vi "AOD Control - debugging(host).vi"() -> ()   [LabVIEW 2009]
uses:
  <vilib>/userdefined/High Color/nirio_resource_hc.ctl
  <vilib>/rvi/interface/nirviOpenFPGA/nirviOpenFPGA.xnode
  FPGA Bitfiles/AOD Control.lvproj_FPGA Target_AOD Control (FPGA)~D2.lvbitx
  AOD Control (FPGA).vi
  <vilib>/rvi/interface/RandomDataEmulation/nirviRandomDataOpen.vi
  <vilib>/rvi/interface/nirviOpenFPGA/nirviOpenFPGA.ctl
  <vilib>/rvi/interface/nirviOpenFPGA/nirviopenstate.ctl
  <vilib>/picture/picture.llb/imagedata.ctl
  <vilib>/rvi/interface/common/nirviIntfCommonState.ctl
  <vilib>/rvi/interface/common/nirviIntfModes.ctl
  C:/Program Files/National Instruments/LabVIEW 2009/resource/RVI/emulation/niLvFpgaEmulationMode.ctl
  <vilib>/eio/XNode/Errors/EIOXNodeErrorStruct.ctl
  <vilib>/eio/XNode/Errors/EIOXNodeInternalErrorTypes.ctl
  <vilib>/eio/XNode/Errors/EIOXNodeUserErrorTypes.ctl
  <vilib>/XNodeSupport/XNodeRect32.ctl
  <vilib>/XNodeSupport/XNodeInt.ctl
  <vilib>/XNodeSupport/XNodeTerms.ctl
  <vilib>/XNodeSupport/XNodeTerm.ctl
  <vilib>/XNodeSupport/XNodeString.ctl
  <vilib>/XNodeSupport/XNodeVariant.ctl
  <vilib>/XNodeSupport/XNodeBool.ctl
  <vilib>/rvi/interface/nirviMethod/nirviMethod.xnode
  <vilib>/FPGA/interface/niFpgaViExecutionMode.ctl
  <vilib>/rvi/errors/niLvFpgaMergeErrorWithErrorCode.vi
  <vilib>/rvi/interface/RandomDataEmulation/nirviRandomDataRunMethod.vi
  <vilib>/rvi/interface/RandomDataEmulation/nirviRandomDataDMAMethods.vi
  <vilib>/rvi/interface/common/niFpgaNodeNameForErrorReporting.ctl
  <vilib>/rvi/interface/nirviReadWriteControl/nirviReadWriteControl.xnode
  <vilib>/Waveform/DWDTOps.llb/DWDT Binary U16 to Digital.vi
  <vilib>/XNodeSupport/NI_XNodeSupport.lvlib
panel:
  in  "TriggerAcq":bool=TRUE
  out "State":T1(ring)
  out "SerialError":bool
  in  "Abort":bool
  out "Acquire":bool
  out "SampleCount":i16
  in  "AcqDivider":i32=10
  in  "Downsample":i32=160
  in  "Reset":bool
  in  "SclkDivider":u32=40
  in  "Pause":u32
  in  "P":bool
  in  "Volume Scan":bool
  in  "Scan Settings":T2={"XStart"=-200000000, "XEnd"=200000000, "XInc"=20000000, "YStart"=-200000000, "YEnd"=200000000, "YInc"=20000000, "ZStart"=-40000, "ZEnd"=40000, "ZInc"=400}
  out "PointTime":u32
  out "NumReps":i32
  out "NumPoints":i32
  out "Read Point":cluster{"X":i32, "Y":i32, "Z":i32}
  out "PointNum":u32
  out "Sequencing error":bool
  out "Count":i32
  in  "Points":i32[][](array[numeric])
  in  "Scans":i32
  in  "Scan":bool
  out "Write count":i32
  out "Written":cluster{"Address":u8, "Value":u32}[](array[cluster]) {"Address" format="%x"; "Value" format="%x"}
  in  "Write Point":bool
  in  "Write Registers":cluster{"Address":u8, "Value":u32}[](array[cluster])=[{"Address"=0, "Value"=240}, {"Address"=1, "Value"=13762592}, {"Address"=2, "Value"=32768}, {"Address"=3, "Value"=8413952}, {"Address"=4, "Value"=0}, {"Address"=5, "Value"=0}, {"Address"=6, "Value"=1023}, {"Address"=7, "Value"=257}, {"Address"=8, "Value"=21}, {"Address"=0, "Value"=246}] {"Address" format="%x"; "Value" format="%x"}
  in  "UpdatesPerPoint":u32=2000
  in  "Write Point":cluster{"X":i32, "Y":i32, "Z":i32}
  in  "Samples":u32=1000
  in  "WriteSize":enum16{"1", "2", "4"}(ring)
  in  "Loopback delay":u32=4
  out "ControlSignals":digitalwaveform(graph)
  out "Elements Remaining":u32
  in  "Stop":bool
  in  "Write Register":bool
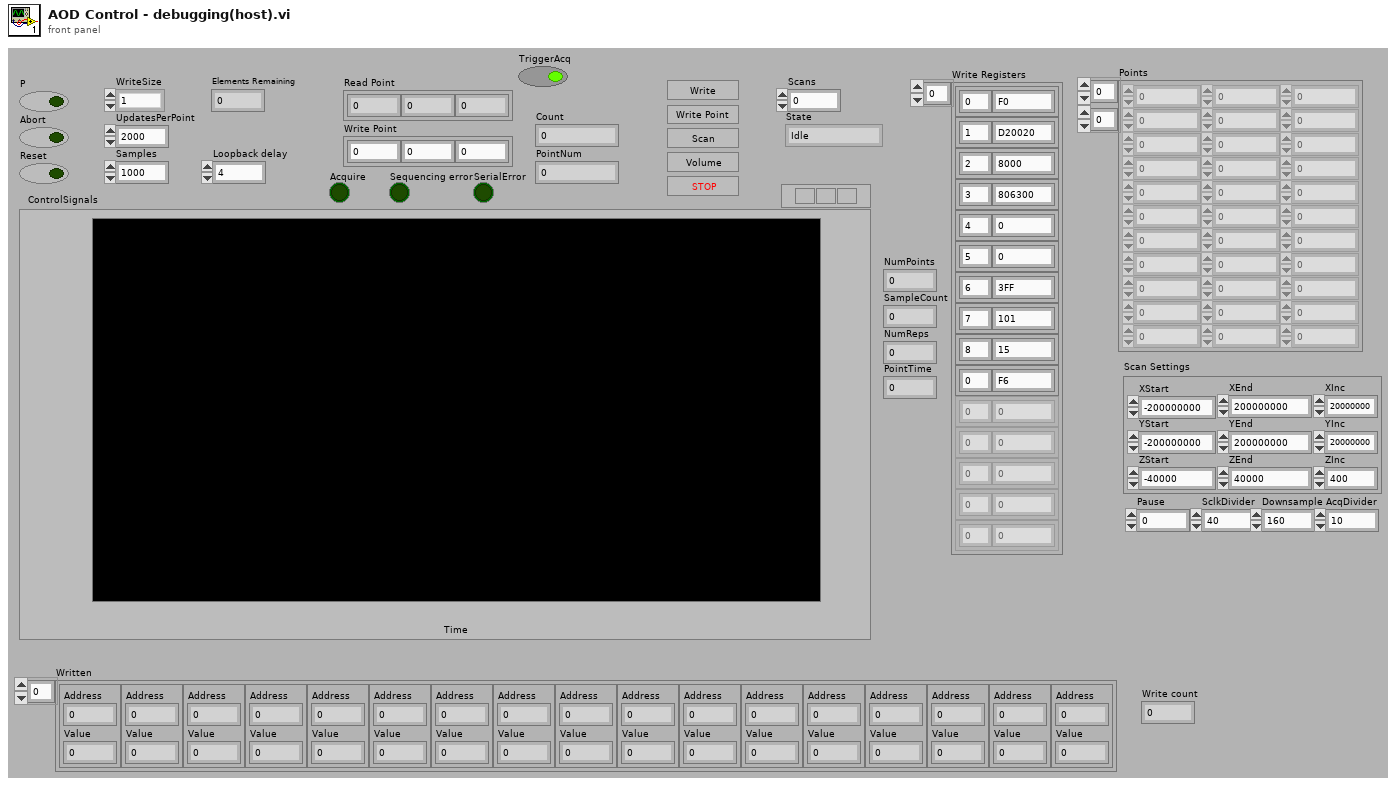
[diagram p1: front panel]
types:
  T1 = enum16{"Idle", "Write Registers", "Receive Points", "Prepare Volume", "Arm Scan", "Scan Points"}
  T2 = cluster{"XStart":i32, "XEnd":i32, "XInc":i32, "YStart":i32, "YEnd":i32, "YInc":i32, "ZStart":i32, "ZEnd":i32, "ZInc":i32}
  T3 = typedef "nirio_resource_hc.ctl" = tag
  T4 = typedef "niFpgaViExecutionMode.ctl" = enum16{"FPGA Target", "Development Computer with Simulated I/O", "Development Computer with Real I/O"}
  T5 = enum16{"Idle", "Write Registers", "Receive Points", "Scan Points"}
  T6 = typedef "niFpgaNodeNameForErrorReporting.ctl" = enum16{"Open FPGA VI Reference", "Read/Write Control", "Invoke Method: Abort", "Invoke Method: Acknowledge IRQ", "Invoke Method: Download", "Invoke Method: FIFO.Configure", "Invoke Method: FIFO.Read", "Invoke Method: FIFO.Start", "Invoke Method: FIFO.Stop", "Invoke Method: FIFO.Write", "Invoke Method: Reset", "Invoke Method: Run", "Invoke Method: Wait on IRQ", "Close FPGA VI Reference"}
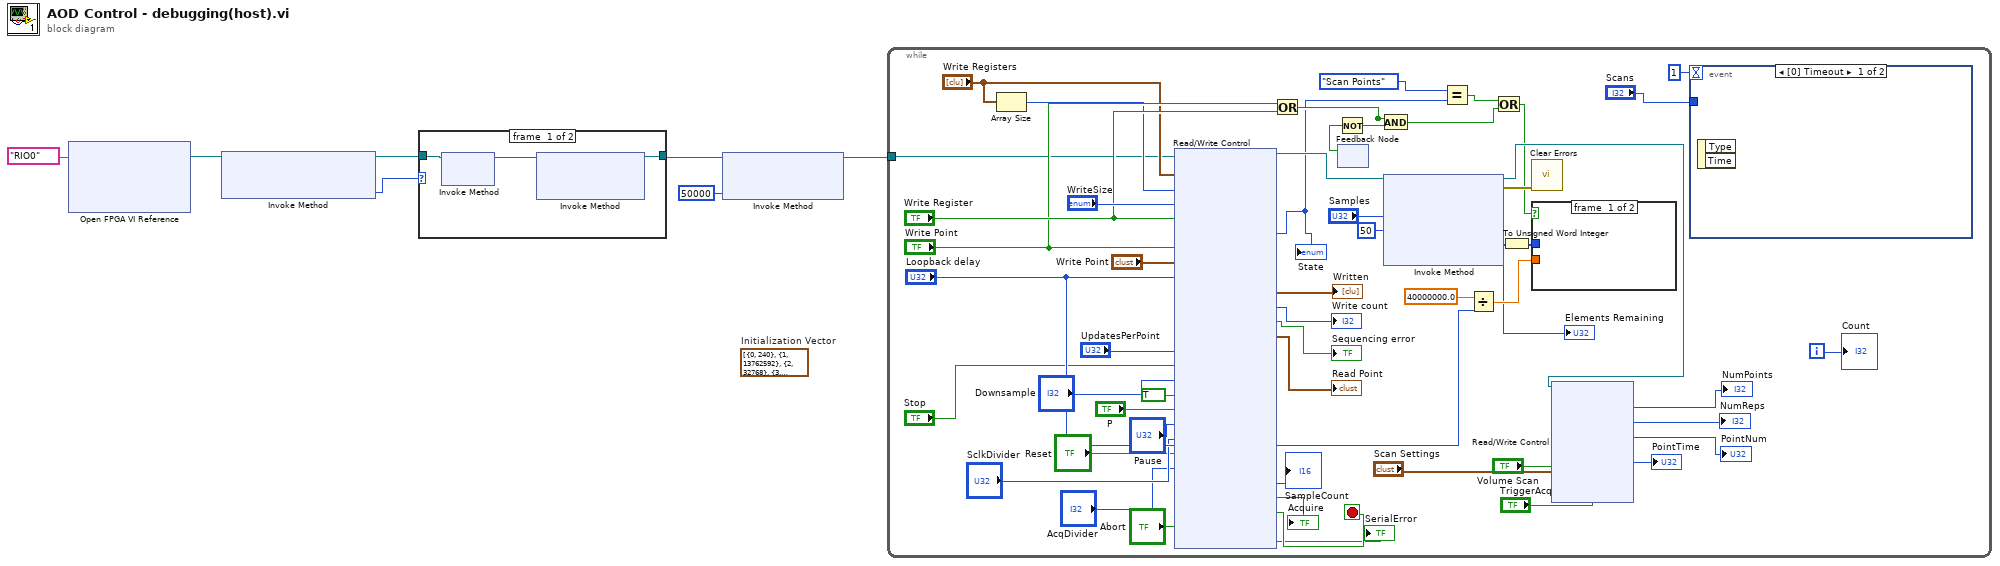
[diagram p0: block diagram]
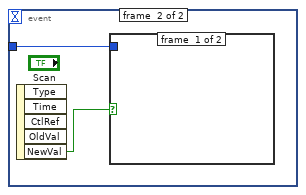
[diagram p3: hidden frame]
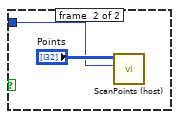
[diagram p4: hidden frame]
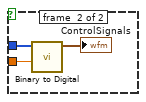
[diagram p5: hidden frame]
diagram:
  (unwired) cluster{"Address":u8, "Value":u32}[] [{"Address"=0, "Value"=240}, {"Address"=1, "Value"=13762592}, {"Address"=2, "Value"=32768}, {"Address"=3, "Value"=8413952}, {"Address"=4, "Value"=0}, {"Address"=5, "Value"=0}, {"Address"=6, "Value"=1023}, {"Address"=7, "Value"=257}, {"Address"=8, "Value"=21}, {"Address"=0, "Value"=246}]  # Initialization Vector
  n1 = xnode "Open FPGA VI Reference"("resource name"=T3 "RIO0") -> ("FPGA VI Reference Out"=w4:refnum<k20>)  [unwired: 1 in, 1 out]
  n2 = xnode "Invoke Method"("FPGA VI Reference In"=w4) -> ("FPGA VI Reference Out"=w2:refnum<k20>, "FPGA VI Execution Mode"=w3:T4)  [unwired: 1 in, 1 out]
  n3 = case shown="\"FPGA Target\", Default" w3 {
    tunnel: [w8 w24] -> w5
    tunnel: w2 -> [w9 w24]
    frame #0 {
      n4 = xnode "Invoke Method"("FPGA VI Reference In"=w9) -> ("FPGA VI Reference Out"=w10:refnum<k20>)  [unwired: 1 in, 1 out]
      n5 = xnode "Invoke Method"("FPGA VI Reference In"=w10) -> ("FPGA VI Reference Out"=w8:refnum<k20>)  [unwired: 2 in, 1 out]
    }
    frame #1 {
    }
  }
  n6 = xnode "Invoke Method"("FPGA VI Reference In"=w5, "Depth"=u32 50000) -> ("FPGA VI Reference Out"=w6:refnum<k20>)  [unwired: 1 in, 1 out]
  n7 = while {
    tunnel: w6 -> [w61]
    i -> [w60]
    stop <- w30 stop-if-true
    n8 = Array Size(array="Write Registers") -> (size(s)=w64:i32)
    n9 = xnode "Read/Write Control"("FPGA VI Reference In"=w61, "Register Writes"="Write Registers", "Number Registers"=w64, "WriteSize"="WriteSize", "Write Register"="Write Register", "Write Point"="Write Point", "Point"="Write Point", "Loopback delay"="Loopback delay", "UpdatesPerPoint"="UpdatesPerPoint", "stop"="Stop", "Downsample"="Downsample", "Loopback"=TRUE, "P"="P", "Pause"="Pause", "SclkDivider"="SclkDivider", "Reset"="Reset", "AcqDivider"="AcqDivider", "Abort"="Abort") -> ("FPGA VI Reference Out"=w70:refnum<k20>, "State"=w27:T1, "Written"=→"Written":cluster{"Address":u8, "Value":u32}[], "Write count"=→"Write count":i32, "Sequencing error"=→"Sequencing error":bool, "Point"=→"Read Point":cluster{"X":i32, "Y":i32, "Z":i32}, "SampleCount"=→"SampleCount":u32, "Acquire"=→"Acquire":bool, "Stopped"=w30:bool, "SerialError"=→"SerialError":bool)  [unwired: 1 in, 1 out]
    "State" <- w27
    n10 = Or(x="Write Point", y="Write Register") -> (x .or. y?=w68:bool)
    n11 = feedback #1() -> (w72:bool)  [unwired: 1 in]
    n12 = Not(x=w72) -> (.not. x?=w71:bool)
    n13 = And(x=w68, y=w71) -> (x .and. y?=w35:bool)
    n14 = xnode "Invoke Method"("FPGA VI Reference In"=w70, "Number of Elements"="Samples", "Timeout (ms)"=50) -> ("FPGA VI Reference Out"=w50:refnum<k20>, "error out"=w77:errorcluster, "Data"=w56:i32[], "Elements Remaining"=→"Elements Remaining":u32)  [unwired: 1 in]
    n15 = Equal?(x=T5."Scan Points" ("State"), y=w27) -> (x = y?=w36:bool)
    n16 = Divide(x=40000000.0, y="Loopback delay") -> (x/y=w76:dbl)
    n17 = Or(x=w36, y=w35) -> (x .or. y?=w34:bool)
    n18 = To Unsigned Word Integer(number=w56) -> (unsigned 16bit integer=w55:u16[])
    n19 = call <vilib>:"Clear Errors.vi"("error in (no error)"=w77) -> ()  [unwired: 6 in, 1 out]
    n20 = case shown="True" w34 {
      tunnel: w55 -> [_ w141]
      tunnel: w76 -> [_ w140]
      frame #0 {
      }
      frame #1 {
        n21 = call-poly <vilib>:"Binary to Digital.vi"("sample rate"=w140, "binary array"=w141) -> ("digital waveform"=→"ControlSignals":digitalwaveform)  [unwired: 8 in, 1 out]
      }
    }
    n22 = xnode "Read/Write Control"("FPGA VI Reference In"=w50, "Volume Scan"="Volume Scan", "Scan Settings"="Scan Settings", "TriggerAcq"="TriggerAcq") -> ("NumPoints"=→"NumPoints":i32, "NumReps"=→"NumReps":i32, "PointNum"=→"PointNum":i32, "PointTime"=→"PointTime":u32)  [unwired: 1 in, 2 out]
    n23 = event shown="[0] Timeout" {
      selector: _ -> [_ _]
      dyn-events: _ -> [_ _]
      timeout: 1 -> [_ _]
      tunnel: "Scans" -> [_ w136]
      event #0 {
        n24 = event-data() -> ()  [unwired: 1 in, 2 out]
      }
      event #1 {
        n25 = event-data() -> ("NewVal"=w137:bool)  [unwired: 1 in, 4 out]
        n26 = case shown="True" w137 {
          tunnel: w136 -> [_ w138]
          frame #0 {
          }
          frame #1 {
            n27 = call "ScanPoints (host).vi"("Scans"=w138, "Points"="Points") -> ()  [unwired: 10 in]
          }
        }
      }
    }
    "Count" <- w60
  }
